vi "SMTP Email Send Message (Small).vi"(5 "return address":string, 6 "strip high bit (T)":bool=TRUE, 7 "mail server":string, 8 "error in (no error)":errorcluster, 9 "message":string, 10 "subject ([No Subject])":string="[No Subject]", 11 "recipient":string) -> (0 "error out":errorcluster)   [LabVIEW 2011, in "NewNI_SMTPEmail.lvlib"]
doc: "Sends a text email to a single recipient. You can use this VI only with ASCII characters."
uses:
  NewNI_SMTPEmail.lvlib
panel:
  out "?":string
  out "?":string
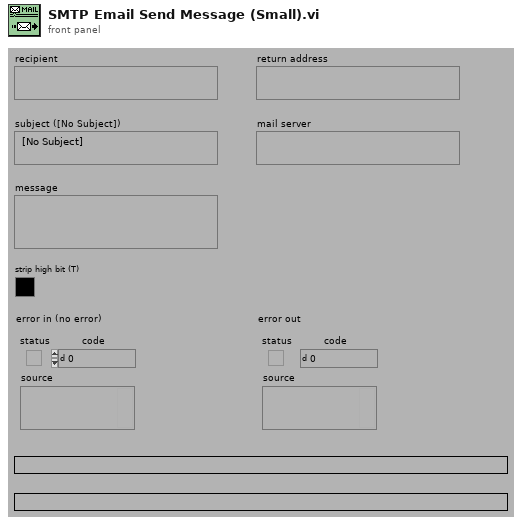
[diagram p1: front panel]
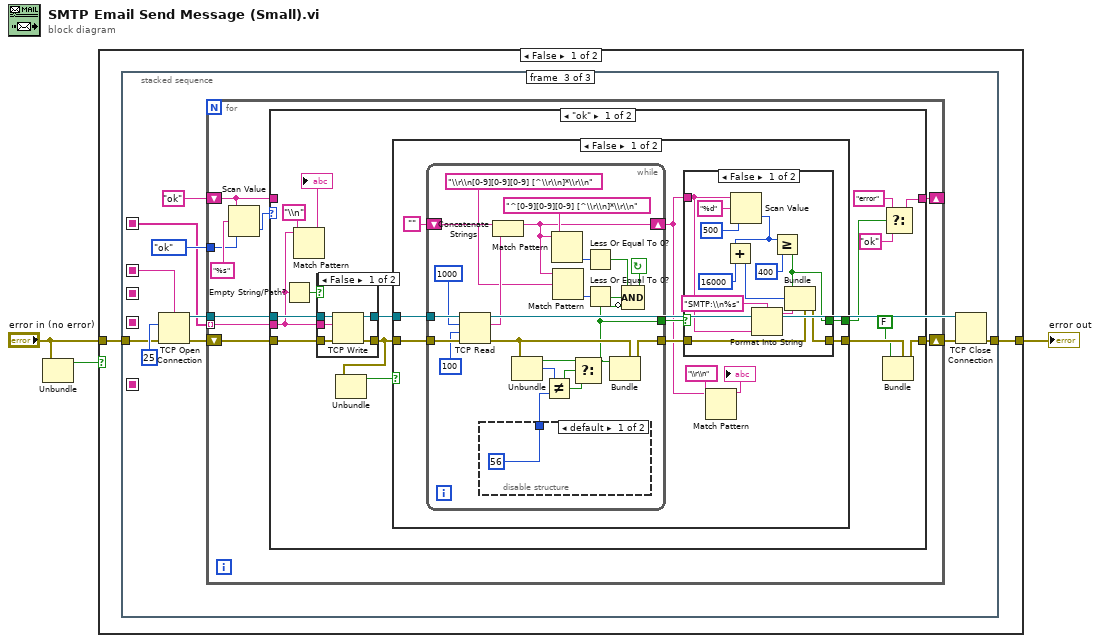
[diagram p0: block diagram]
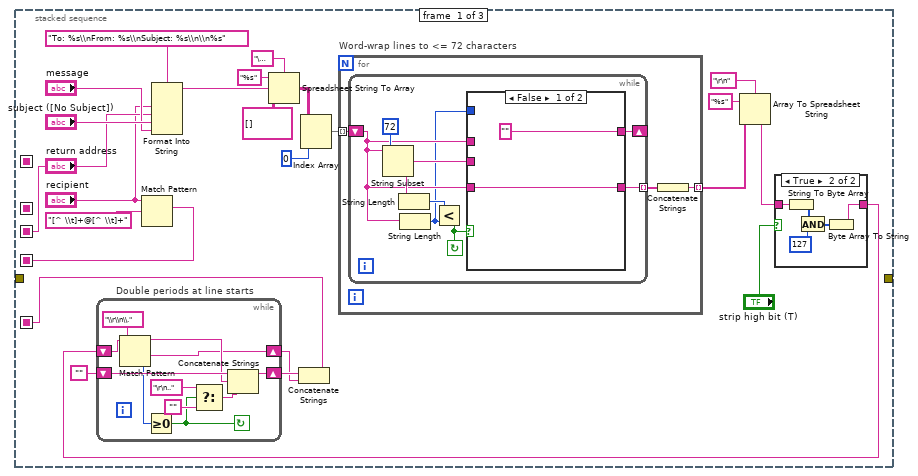
[diagram p2: hidden frame]
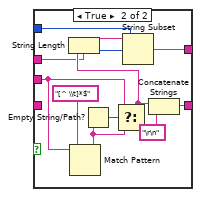
[diagram p4: hidden frame]
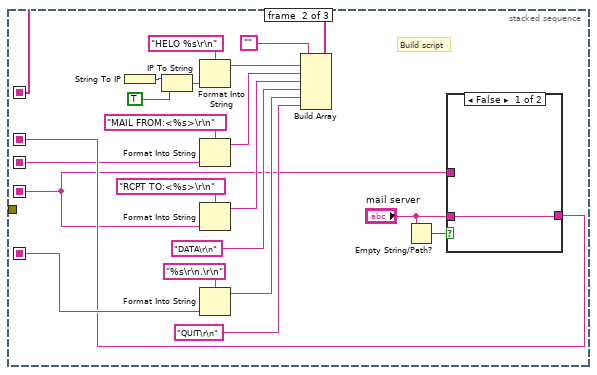
[diagram p5: hidden frame]
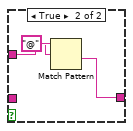
[diagram p6: hidden frame]
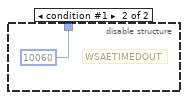
[diagram p8: hidden frame]
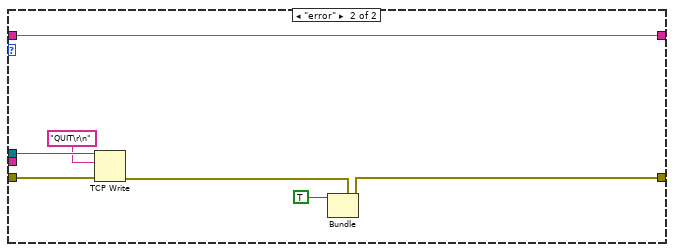
[diagram p11: hidden frame]
diagram:
  n1 = Unbundle("error in (no error)") -> ("status"=w1:bool)  [unwired: 2 out]
  n2 = case shown="False" w1 {
    tunnel: "error in (no error)" -> [w5 w194]
    tunnel: [w4 w194] -> w3
    frame False {
      n3 = stacked-sequence {
        seq-local: [_ w77 _] -> [_ _ w98]
        seq-local: ["return address" _ _] -> [_ w72 _]
        seq-local: [w6 _ _] -> [_ w71 _]
        seq-local: [w9 _ _] -> [_ w76 _]
        seq-local: [_ w73 _] -> [_ _ w96]
        tunnel: [_ _ w105] -> w4
        tunnel: w5 -> [_ _ w97]
        frame #0 {
          n4 = Match Pattern(string="recipient", regular expression="[^ \\t]+@[^ \\t]+") -> (match substring=w6:string)  [unwired: 4 out]
          n5 = Format Into String(format string="To: %s\\nFrom: %s\\nSubject: %s\\n\\n%s", "recipient", "return address", "subject ([No Subject])", "message") -> (resulting string=w19:string)  [unwired: 2 in, 1 out]
          n6 = Spreadsheet String To Array(delimiter (Tab)="\u0000", format string="%s", spreadsheet string=w19, array type (2D Dbl)=string[][] []) -> (array=w25:string[][])
          n7 = Index Array(array=w25, index (col)=0) -> (element=w22:string[])  [unwired: 1 in]
          n8 = for "Word-wrap lines to <= 72 characters" {
            tunnel: w22 -> [w49] mode=indexing
            tunnel: [w47] -> w21 mode=indexing
            n9 = while {
              tunnel: [w54] -> w48 mode=indexing
              shift-left: w49 -> [w53]
              shift-right: [w51] -> _
              stop <- w50 continue-if-true
              n10 = String Subset(string=w53, length (rest)=72 ("length")) -> (substring=w56:string)  [unwired: 1 out]
              n11 = String Length(string=w56) -> (length=w55:i32)
              n12 = String Length(string=w53) -> (length=w52:i32)
              n13 = Less?(x=w55, y=w52) -> (x < y?=w50:bool)
              n14 = case shown="False" w50 {
                tunnel: w56 -> [_ w60]
                tunnel: w53 -> [w59 _]
                tunnel: [w59 w64] -> w54
                tunnel: w53 -> [_ w61]
                tunnel: w52 -> [_ w68]
                tunnel: ["" ("substring") w67] -> w51
                frame False {
                }
                frame True {
                  n15 = Match Pattern(string=w60, regular expression="[^ \\t]*$") -> (before substring=w65:string)  [unwired: 4 out]
                  n16 = Empty String/Path?(string/path=w65) -> (empty?=w66:bool)
                  n17 = Select(t=w60, s=w66, f=w65) -> (s? t:f=w63:string)
                  n18 = String Length(string=w63) -> (length=w69:i32)
                  n19 = String Subset(string=w61, offset (0)=w69, length (rest)=w68) -> (substring=w67:string)
                  n20 = Concatenate Strings(w63, "\r\n" ("delimiter (Tab)")) -> (w64:string)
                }
              }
            }
            n21 = Concatenate Strings(w48) -> (w47:string)
          }
          n22 = Array To Spreadsheet String(delimiter (Tab)="\r\n", array=w21, 3:"%s" ("format string")) -> (spreadsheet string=w15:string)
          n23 = case shown="True" "strip high bit (T)" {
            tunnel: [w41 w42] -> w10
            tunnel: w15 -> [w41 w46]
            frame False {
            }
            frame True {
              n24 = String To Byte Array(string=w46) -> (unsigned byte array=w43:u8[])
              n25 = And(x=w43, y=u8 127) -> (x .and. y?=w45:u8[])
              n26 = Byte Array To String(unsigned byte array=w45) -> (string=w42:string)
            }
          }
          n27 = while "Double periods at line starts" {
            shift-left: w10 -> [w34]
            shift-right: [w33] -> w11
            shift-left: "" -> [w40]
            shift-right: [w39] -> w12
            stop <- w30 continue-if-true
            n28 = Match Pattern(string=w34, regular expression="\\r\\n\\.") -> (before substring=w38:string, after substring=w33:string, offset past match=w37:i32)  [unwired: 2 out]
            n29 = Greater Or Equal To 0?(x=w37) -> (x >= 0?=w30:bool)
            n30 = Select(t="\r\n.." ("regular expression"), s=w30, f="") -> (s? t:f=w36:string)
            n31 = Concatenate Strings(w40, w38, w36) -> (w39:string)
          }
          n32 = Concatenate Strings(w12, w11) -> (w9:string)
        }
        frame #1 {
          # "Build script"
          n33 = String To IP() -> (0:w81:u32)  [unwired: 1 out]
          n34 = IP To String(1:TRUE ("dot notation? (F)"), 2:w81) -> (0:w79:string)
          n35 = Format Into String(format string="HELO %s\r\n", w79) -> (resulting string=w82:string)  [unwired: 2 in, 1 out]
          n36 = Format Into String(format string="MAIL FROM:<%s>\r\n", w72) -> (resulting string=w85:string)  [unwired: 2 in, 1 out]
          n37 = Format Into String(format string="RCPT TO:<%s>\r\n", w71) -> (resulting string=w87:string)  [unwired: 2 in, 1 out]
          n38 = Format Into String(format string="%s\r\n.\r\n", w76) -> (resulting string=w90:string)  [unwired: 2 in, 1 out]
          n39 = Build Array("", w82, w85, w87, "DATA\r\n", w90, "QUIT\r\n") -> (w77:string[])
          n40 = Empty String/Path?(string/path="mail server") -> (empty?=w75:bool)
          n41 = case shown="False" w75 {
            tunnel: w71 -> [_ w95]
            tunnel: [w92 w93] -> w73
            tunnel: "mail server" -> [w92 _]
            frame False {
            }
            frame True {
              n42 = Match Pattern(string=w95, regular expression="@") -> (after substring=w93:string)  [unwired: 4 out]
            }
          }
        }
        frame #2 {
          n43 = TCP Open Connection(address=w96, remote port or service name=u16 25 ("remote port"), error in (no error)=w97) -> (connection ID=w102:refnum<k5>, error out=w99:errorcluster)  [unwired: 2 out]
          n44 = for {
            tunnel: enum16{"ok", "error"}."ok" -> [w113]
            shift-right: [w106] -> w101
            shift-left: w99 -> [w111]
            tunnel: w102 -> [w110]
            shift-right: [w108] -> _
            shift-left: "ok" -> [w109]
            tunnel: w98 -> [w107] mode=indexing
            n45 = Scan Value(string=w109, format string="%s", default (0 dbl)=w113) -> (value=w112:enum16{"ok", "error"})  [unwired: 1 out]
            n46 = case shown="\"ok\"" w112 {
              tunnel: w107 -> [w115 _]
              tunnel: w111 -> [w130 w190]
              tunnel: [w122 w191] -> w106
              tunnel: w110 -> [w129 w189]
              tunnel: [w125 w193] -> w108
              tunnel: w109 -> [_ w193]
              frame "ok" {
                n47 = Empty String/Path?(string/path=w115) -> (empty?=w116:bool)
                n48 = Match Pattern(string=w115, regular expression="\\n") -> (before substring=→"?":string)  [unwired: 4 out]
                n49 = case shown="False" w116 {
                  tunnel: [w135 w136] -> w118
                  tunnel: w115 -> [w134 _]
                  tunnel: [w133 w137] -> w128
                  tunnel: w129 -> [w132 w137]
                  tunnel: w130 -> [w131 w136]
                  frame False {
                    n50 = TCP Write(connection ID=w132, data in=w134, error in (no error)=w131) -> (connection ID out=w133:refnum<k5>, error out=w135:errorcluster)  [unwired: 2 out]
                  }
                  frame True {
                  }
                }
                n51 = Unbundle(w118) -> ("status"=w117:bool)  [unwired: 2 out]
                n52 = case shown="False" w117 {
                  selector: w117 -> [_ w185]
                  tunnel: [w141 w186] -> w123
                  tunnel: [w139 w185] -> w127
                  tunnel: w128 -> [w146 _]
                  tunnel: w118 -> [w145 w186]
                  frame False {
                    n53 = while {
                      tunnel: [w151] -> w140
                      shift-left: "" -> [w164]
                      shift-right: [w149] -> w138
                      tunnel: w145 -> [w167]
                      tunnel: [w157] -> w142
                      tunnel: w146 -> [w168]
                      stop <- w154 continue-if-true
                      n54 = TCP Read(connection ID=w168, bytes to read=1000, error in (no error)=w167, 9:100 ("bytes to read")) -> (data out=w163:string, error out=w158:errorcluster)  [unwired: 2 out]
                      n55 = disable-structure shown="default" {
                        disable-tunnel: [56 ("y") 10060 ("x")] -> w148
                        frame condition #0 (active) {
                        }
                        frame condition #1 {
                          # "WSAETIMEDOUT"
                        }
                      }
                      n56 = Concatenate Strings(w164, w163) -> (w149:string)
                      n57 = Unbundle(w158) -> ("status"=w159:bool, "code"=w161:i32)  [unwired: 1 out]
                      n58 = Not Equal?(x=w161, y=w148) -> (x != y?=w160:bool)
                      n59 = Match Pattern(string=w149, regular expression="^[0-9][0-9][0-9] [^\\r\\n]*\\r\\n") -> (offset past match=w156:i32)  [unwired: 4 out]
                      n60 = Match Pattern(string=w149, regular expression="\\r\\n[0-9][0-9][0-9] [^\\r\\n]*\\r\\n") -> (offset past match=w153:i32)  [unwired: 4 out]
                      n61 = Select(t=w159, s=w160, f=w160) -> (s? t:f=w151:bool)
                      n62 = Less Or Equal To 0?(x=w156) -> (x <= 0?=w155:bool)
                      n63 = Less Or Equal To 0?(x=w153) -> (x <= 0?=w152:bool)
                      n64 = Bundle(cluster=w158, "status"=w151) -> (w157:errorcluster)  [unwired: 2 out]
                      n65 = Compound Arithmetic op=AND(w155, w152, invert w151) -> (w154:bool)
                    }
                    n66 = case shown="False" w140 {
                      selector: w140 -> [_ w183]
                      tunnel: [w177 w184] -> w141
                      tunnel: w142 -> [w178 w184]
                      tunnel: [w175 w183] -> w139
                      tunnel: w138 -> [w173 _]
                      frame False {
                        n67 = Scan Value(string=w173, format string="%d", default (0 dbl)=500 ("bytes to read")) -> (value=w176:i32)  [unwired: 1 out]
                        n68 = Add(x=w176, y=16000) -> (x+y=w179:i32)
                        n69 = Format Into String(format string="SMTP:\\n%s", w173) -> (resulting string=w172:string)  [unwired: 2 in, 1 out]
                        n70 = Greater Or Equal?(x=w176, y=400 ("bytes to read")) -> (x >= y?=w175:bool)
                        n71 = Bundle(cluster=w178, "status"=w175, "code"=w179, "source"=w172) -> (w177:errorcluster)
                      }
                      frame True {
                      }
                    }
                    n72 = Match Pattern(string=w138, regular expression="\\r\\n") -> (before substring=→"?":string)  [unwired: 4 out]
                  }
                  frame True {
                  }
                }
                n73 = Bundle(cluster=w123, "status"=FALSE) -> (w122:errorcluster)  [unwired: 2 out]
                n74 = Select(t="error", s=w127, f="ok") -> (s? t:f=w125:string)
              }
              frame "error" {
                n75 = TCP Write(connection ID=w189, data in="QUIT\r\n", error in (no error)=w190) -> (error out=w188:errorcluster)  [unwired: 3 out]
                n76 = Bundle(cluster=w188, "status"=TRUE) -> (w191:errorcluster)  [unwired: 2 out]
              }
            }
          }
          n77 = TCP Close Connection(connection ID=w102, error in (no error)=w101) -> (error out=w105:errorcluster)  [unwired: 2 out]
        }
      }
    }
    frame True {
    }
  }
  "error out" <- w3
